vi "WeatherReport.vi"() -> ()   [LabVIEW 2016, in "WeatherReport.lvlib"]
doc: "This is a simple weather report which can display information for a particular day. This also has options to configure the properties of the controls"
uses:
  WeatherReport.lvlib
panel:
  in  "Settings":bool
  out "Humidity":string="40 %"
  out "Temperature":string="38°C "
  out "Weather":picture
  in  "Options":i32(listbox)
  in  "Stop":bool
  in  "Properties":string(tree)
  in  "Weather Report":i32(listbox)
  out "error out":errorcluster
  in  "Error In":errorcluster
  # "Overview: Demonstrates a typical weather report and provides options to configure the properties of these controls\nInstructions: \n1.Run the VI\n2.Select a particular day in the weather report\n3.The respective information of the day will be populated in the adjacent controls\n4.Click the settings option to list the configuration options for the controls\n5.Select a particular control's property, the possible options will be populated .\n6.Selecting an option applies the property to the control."
  # "The Properties are used to visualize the available controls and configure the visibility and accessibility of them. Selecting the Options applies the property to that control"
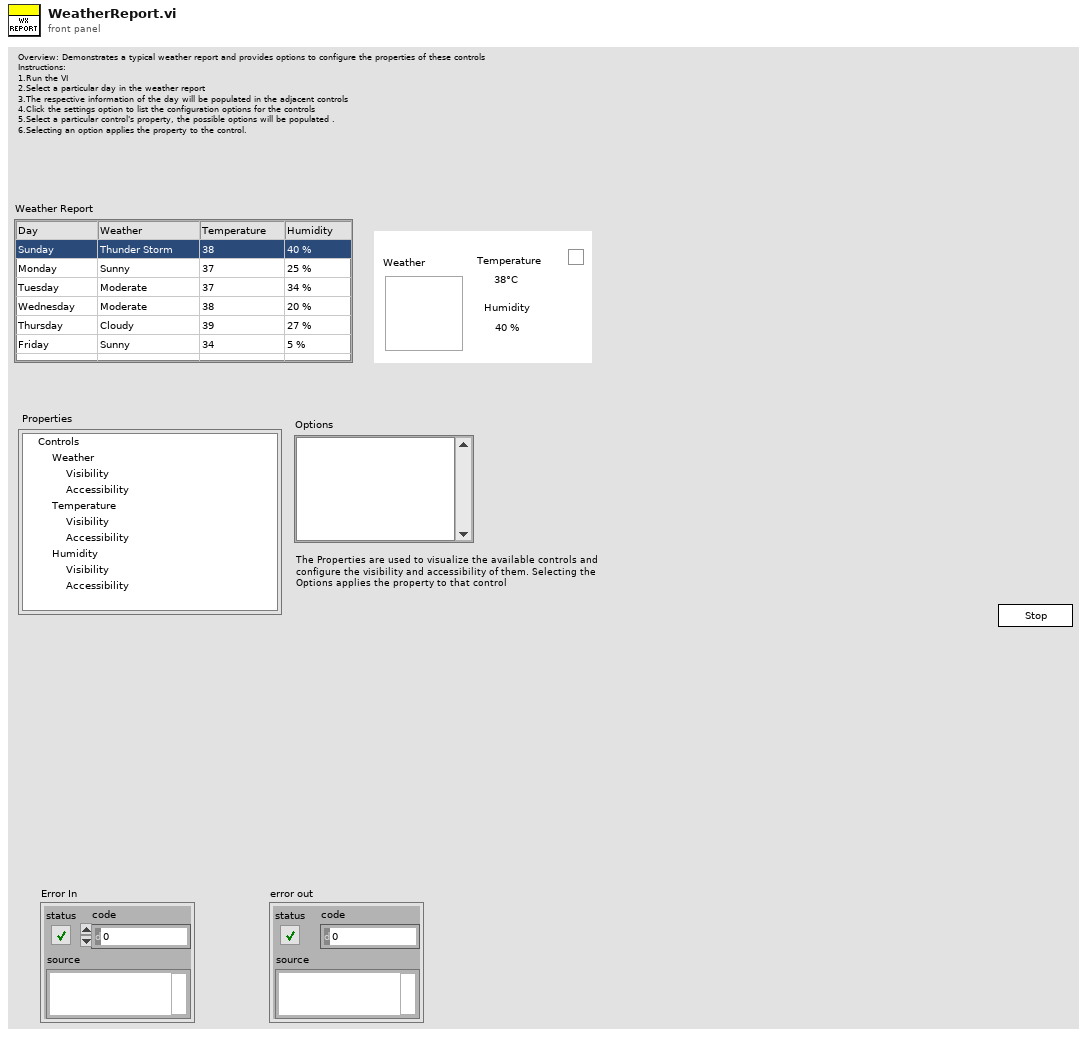
[diagram p1: front panel]
types:
  T1 = cluster{"Left":i16, "Top":i16, "Right":i16, "Bottom":i16}
  T2 = enum32{"Invalid", "Standard", "Closed", "Hidden", "Minimized", "Maximized"}
  T3 = enum32{"invalid app kind", "Development System", "Run Time System", "Student Edition", "Embedded LabVIEW", "Evaluation", "Custom"}
  T4 = enum8{"Enabled", "Disabled", "Disabled and Grayed Out"}
  T5 = enum8{"Enabled", "Disabled", "Disabled and Grayed Out"}[]
  T6 = cluster{"Core":cluster{"Current VI Reference":refnum<vi>, "Close Panel on Exit?":bool}, "Property":string, "Accessibility Array":i32[], "Visibility Array":i32[]}
  T7 = cluster{"Current VI Reference":refnum<vi>, "Close Panel on Exit?":bool}
  T8 = typedef "imagedata.ctl" = cluster{"image type":i32, "image depth":i32, "image":u8[], "mask":u8[], "colors":u32[], "Rectangle":cluster{"left":i16, "top":i16, "right":i16, "bottom":i16}}
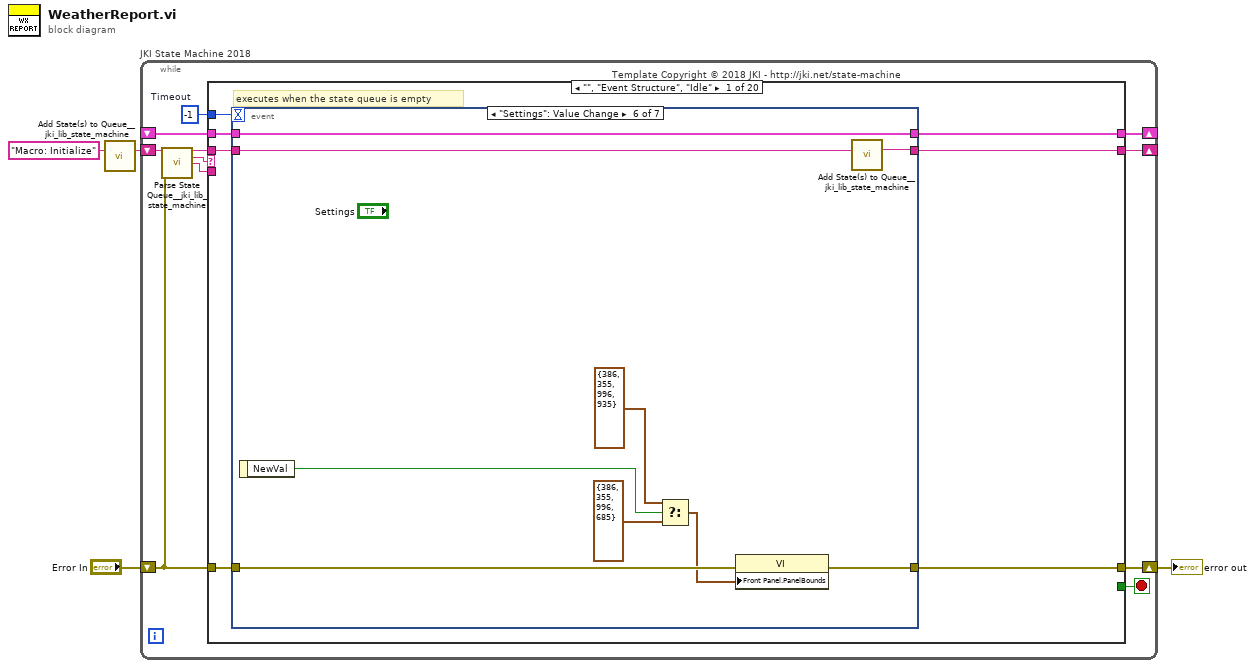
[diagram p0: block diagram]
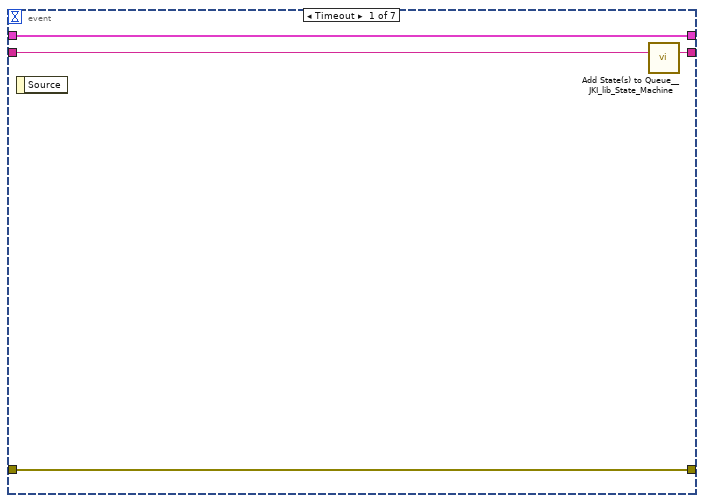
[diagram p2: hidden frame]
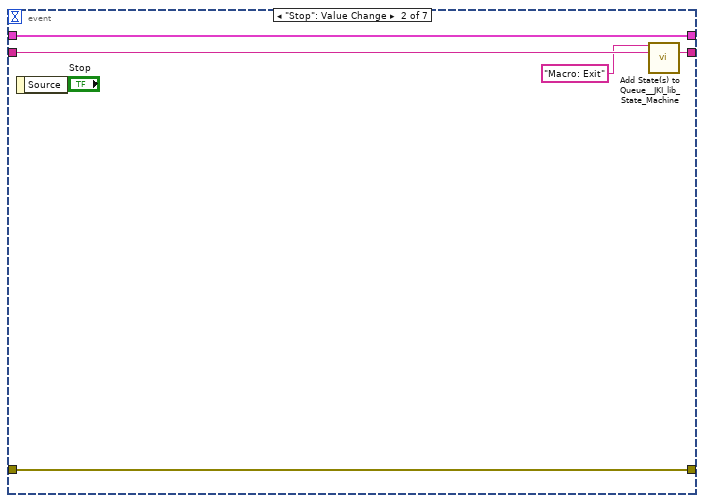
[diagram p3: hidden frame]
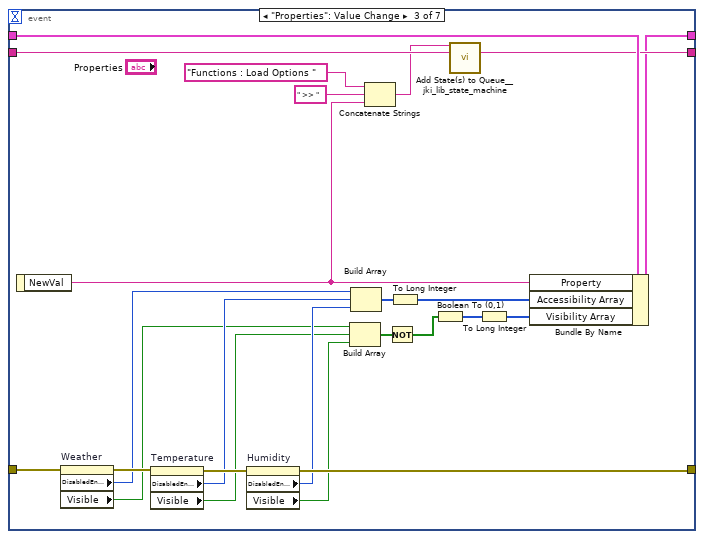
[diagram p4: hidden frame]
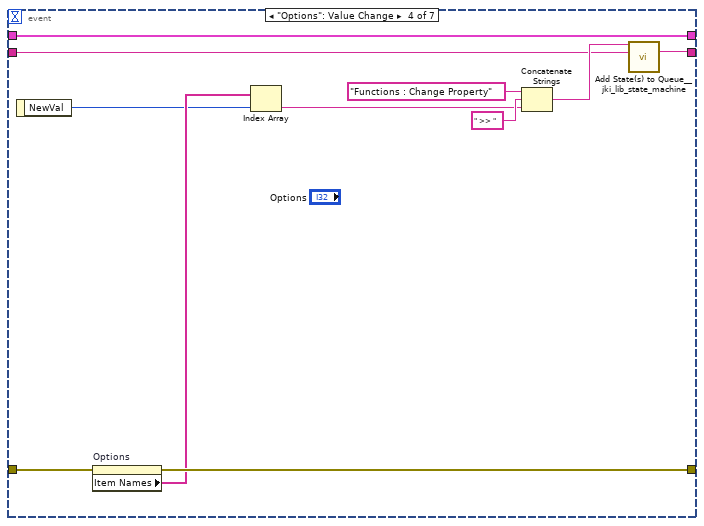
[diagram p5: hidden frame]
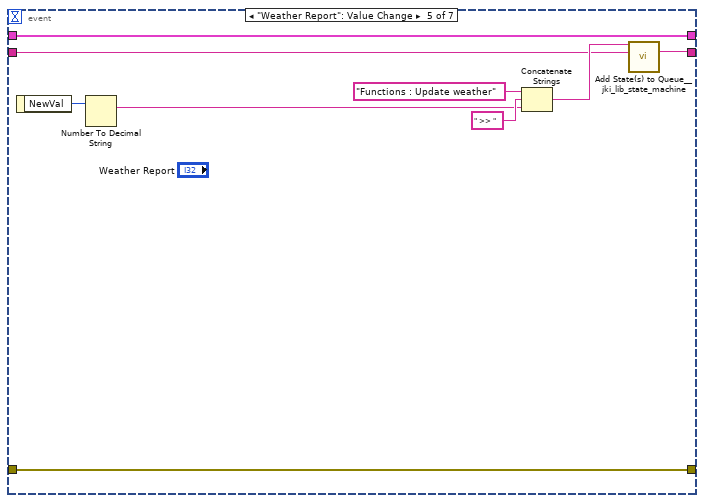
[diagram p6: hidden frame]
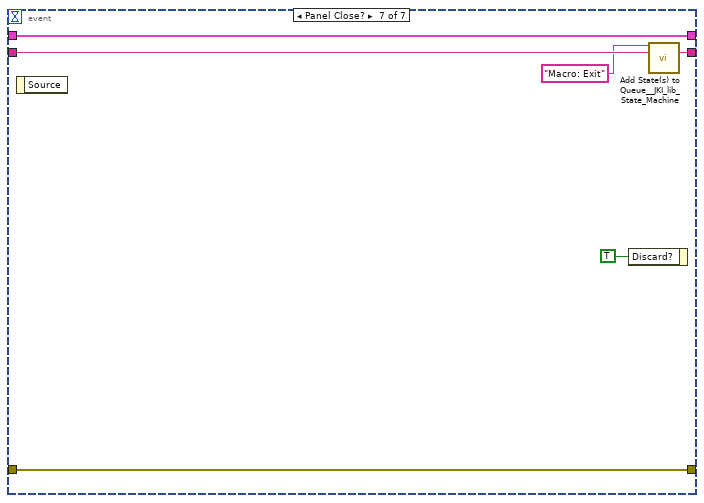
[diagram p7: hidden frame]
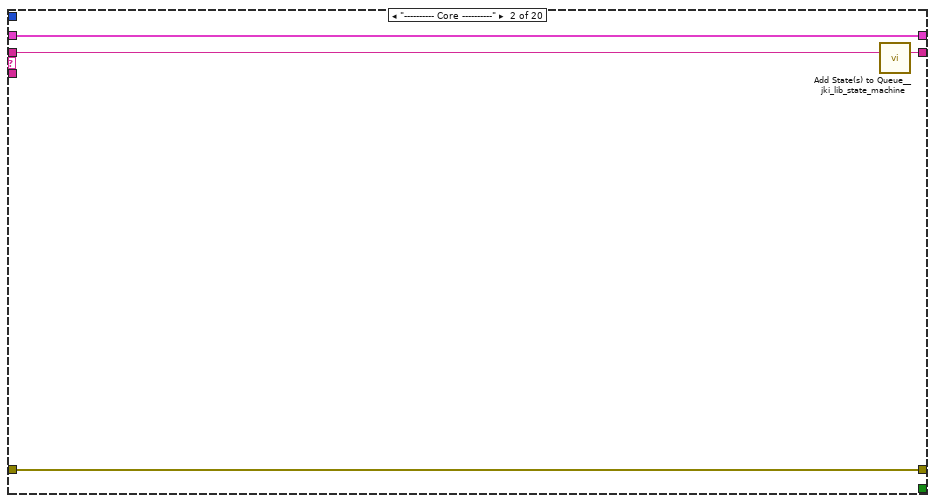
[diagram p8: hidden frame]
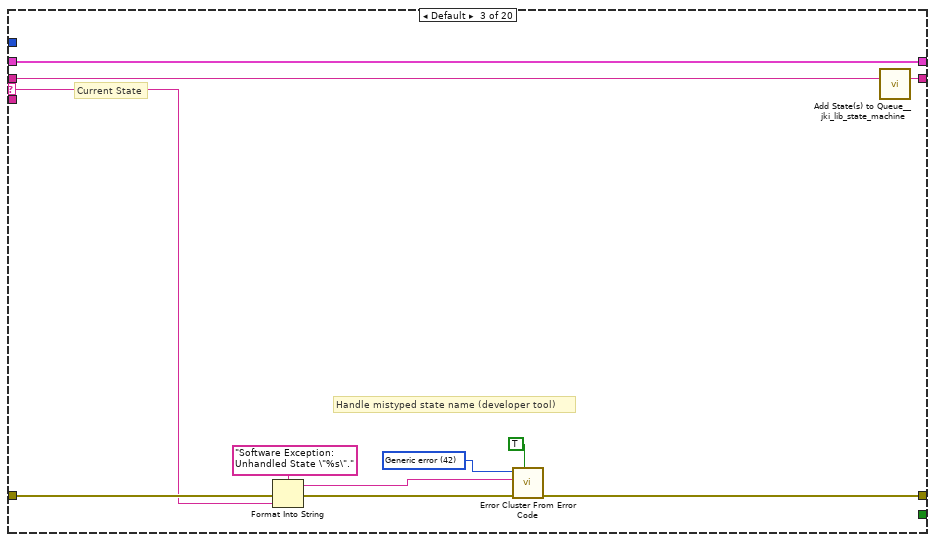
[diagram p9: hidden frame]
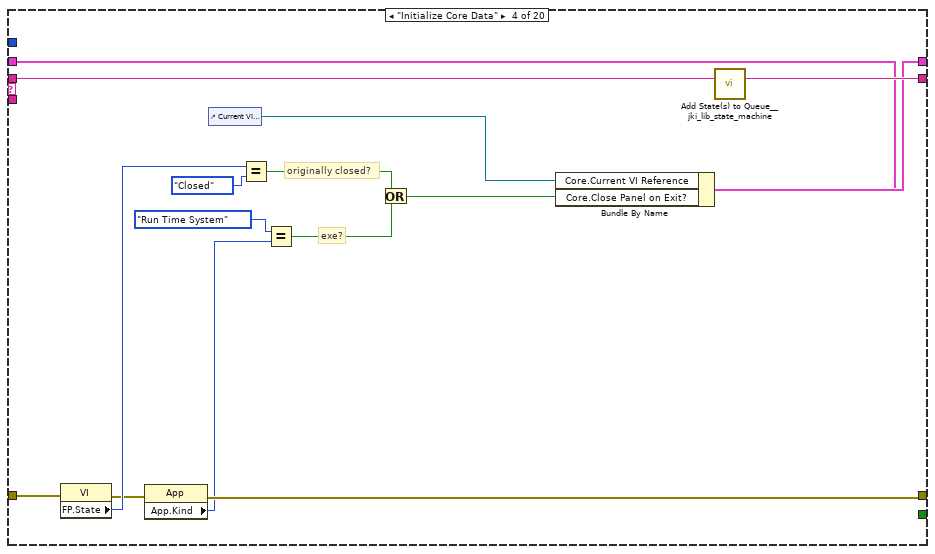
[diagram p10: hidden frame]
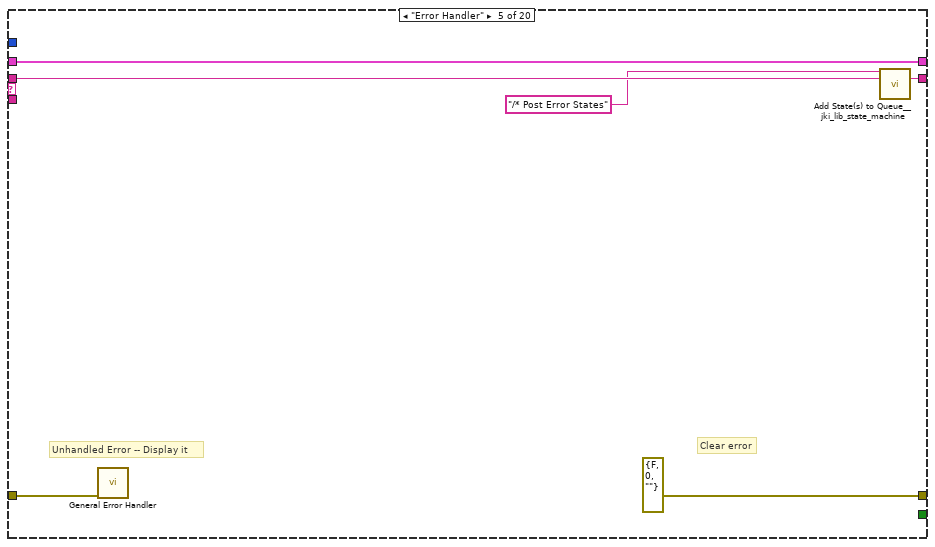
[diagram p11: hidden frame]
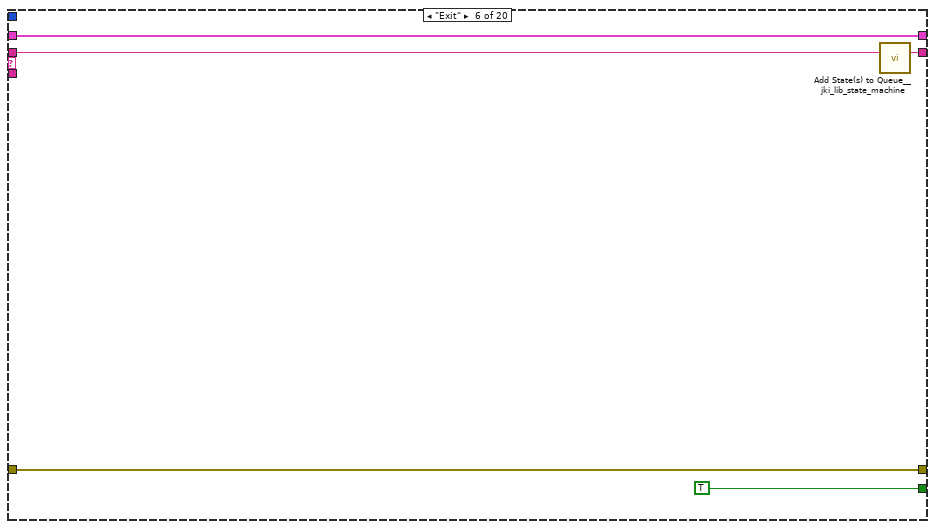
[diagram p12: hidden frame]
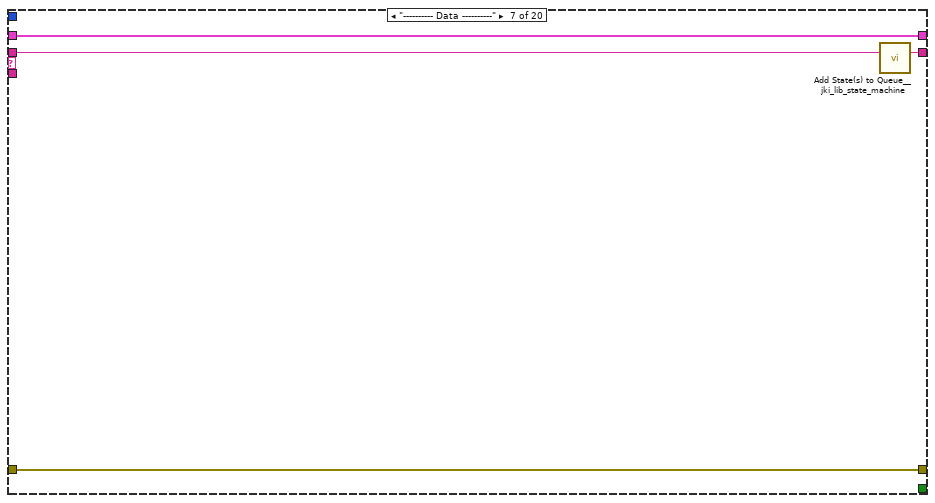
[diagram p13: hidden frame]
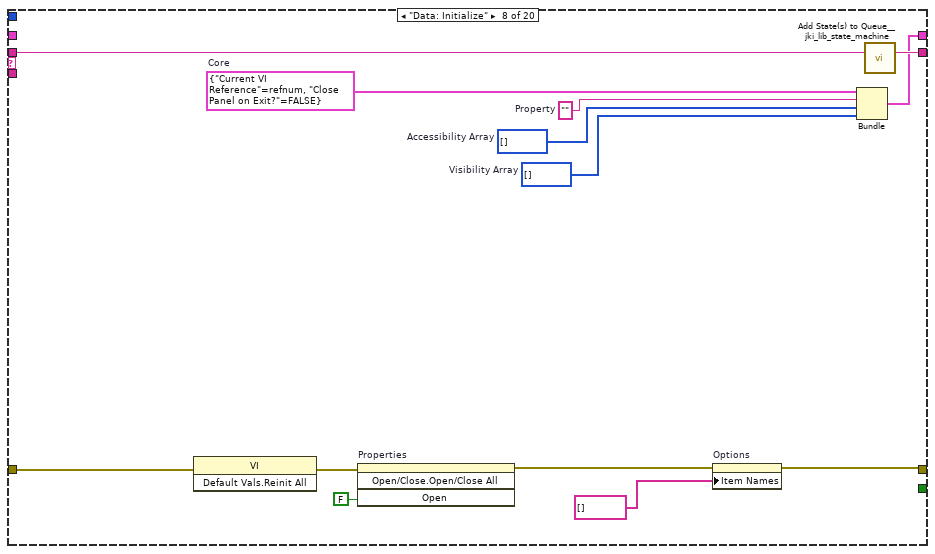
[diagram p14: hidden frame]
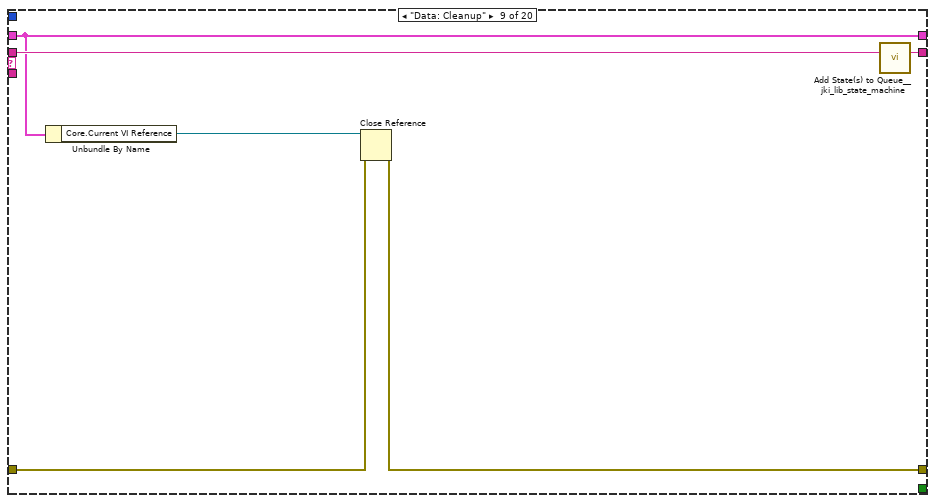
[diagram p15: hidden frame]
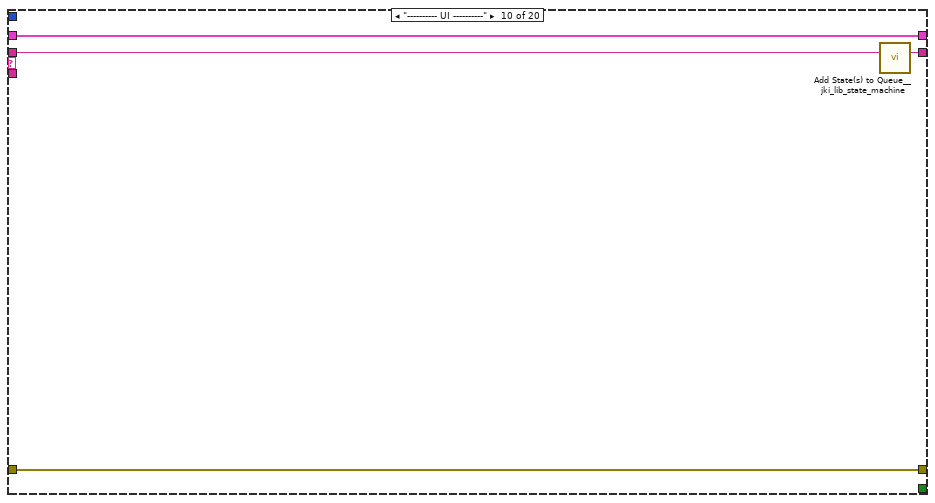
[diagram p16: hidden frame]
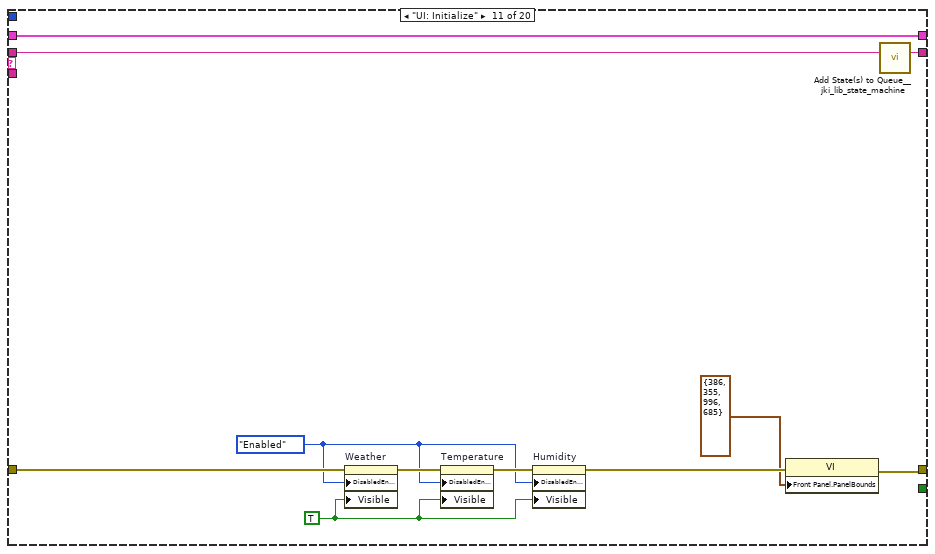
[diagram p17: hidden frame]
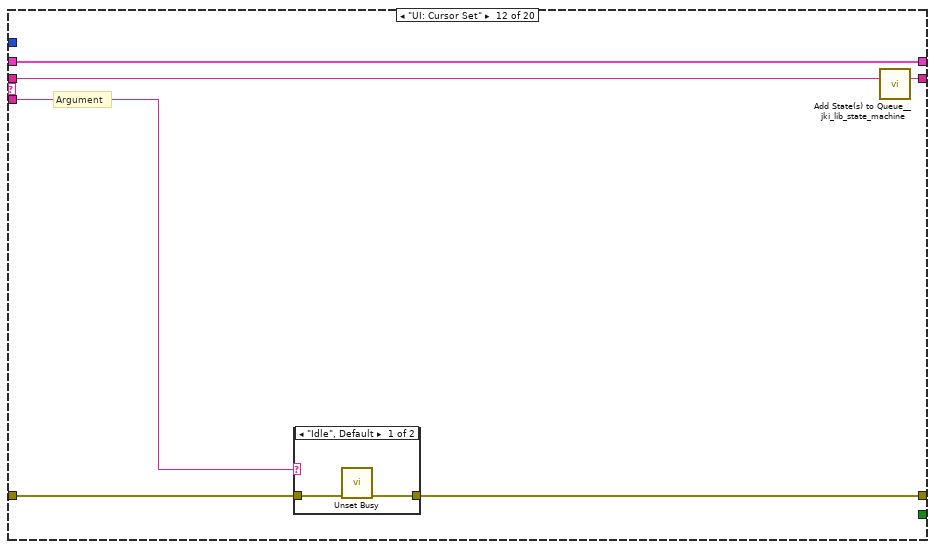
[diagram p18: hidden frame]
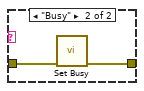
[diagram p19: hidden frame]
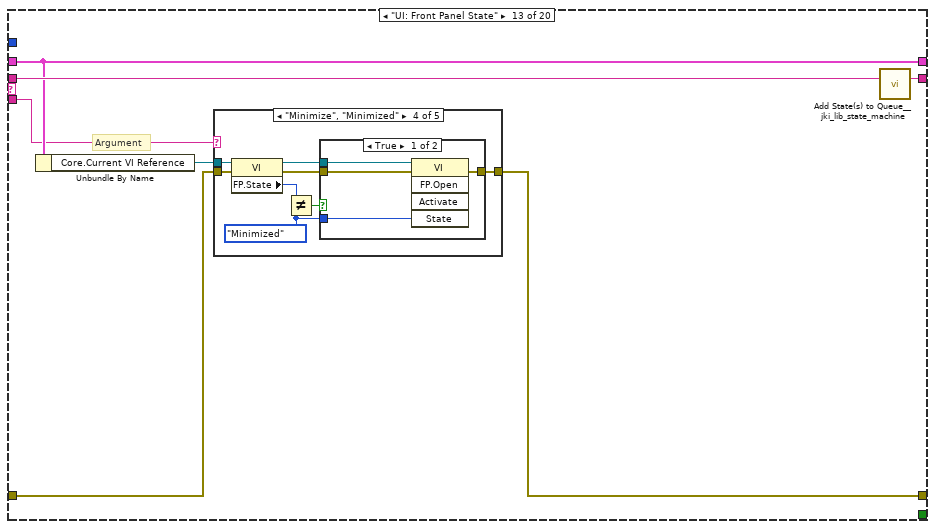
[diagram p20: hidden frame]
diagram:
  n1 = call <vilib>:"Add State(s) to Queue__jki_lib_state_machine.vi"("State(s) in (\"\")"="Macro: Initialize") -> ("States Out"=w4:string)  [unwired: 14 in]
  n2 = while "JKI State Machine 2018" {
    shift-right: [w8] -> _
    shift-left: _ -> [w7]
    shift-right: [w11] -> w1
    shift-left: "Error In" -> [w5]
    shift-right: [w10] -> _
    shift-left: w4 -> [w12]
    stop <- w9 stop-if-true
    w6 = -1  # Timeout
    # "Template Copyright © 2018 JKI - http://jki.net/state-machine"
    n3 = call <vilib>:"Parse State Queue__jki_lib_state_machine.vi"("State Queue"=w12, "Error In (no error)"=w5) -> ("Remaining States"=w14:string, "Current State"=w15:string, "Arguments"=w13:string)  [unwired: 11 in]
    n4 = case shown="\"\", \"Event Structure\", \"Idle\"" w15 {
      selector: w15 -> [_ _ w95 _ _ _ _ _ _ _ _ _ _ _ _ _ _ _ _ _]
      tunnel: w14 -> [w22 w94 w99 w120 w126 w131 w135 w148 w154 w158 w169 w175 w186 w255 w260 w270 w274 w293 w315 w366]
      tunnel: w13 -> [_ _ _ _ _ _ _ _ _ _ _ w170 w180 _ _ _ _ w281 w310 w354]
      tunnel: w7 -> [w20 w91 w97 w116 w123 w129 w132 _ w149 w155 w167 w173 w182 w252 w257 w267 w271 w285 w312 w364]
      tunnel: [w19 w92 w101 w107 errorcluster {"status"=FALSE, "code"=0, "source"=""} ("error out") w128 w133 w137 w150 w156 w163 w171 w183 w253 w258 w268 w272 w290 w303 w359] -> w11
      tunnel: w5 -> [w18 w92 w100 w110 w122 w128 w133 w143 w151 w156 w166 w172 w184 w253 w258 w268 w272 w291 w304 w360]
      tunnel: [w21 w93 w98 w119 w125 w130 w134 w147 w153 w157 w168 w174 w185 w254 w259 w269 w273 w292 w314 w365] -> w10
      tunnel: [_ _ _ _ _ TRUE _ _ _ _ _ _ _ _ _ _ _ _ _ _] -> w9
      tunnel: [w17 w91 w97 w118 w123 w129 w132 w146 w149 w155 w167 w173 w182 w252 w257 w267 w271 w285 w312 w364] -> w8
      tunnel: w6 -> [w16 _ _ _ _ _ _ _ _ _ _ _ _ _ _ _ _ _ _ _]
      frame "", "Event Structure", "Idle" {
        # "executes when the state queue is empty"
        n5 = event shown="[5] \"Settings\": Value Change" {
          selector: _ -> [_ _ _ _ _ _ _]
          dyn-events: _ -> [_ _ _ _ _ _ _]
          timeout: w16 -> [_ _ _ _ _ _ _]
          tunnel: w22 -> [w26 w31 w53 w61 w69 w82 w90]
          tunnel: [w25 w30 w52 w60 w68 w81 w89] -> w21
          tunnel: w20 -> [w23 w28 w54 w65 w74 w83 w87]
          tunnel: [w24 w29 w44 w59 w75 w80 w88] -> w19
          tunnel: w18 -> [w24 w29 w55 w66 w75 w84 w88]
          tunnel: [w23 w28 w48 w65 w74 w83 w87] -> w17
          event Timeout {
            n6 = event-data() -> ()  [unwired: 1 in, 1 out]
            n7 = call <vilib>:"Add State(s) to Queue__JKI_lib_State_Machine.vi"("State(s) in (\"\")"=w26) -> ("States Out"=w25:string)  [unwired: 14 in]
          }
          event "Stop": Value Change {
            n8 = event-data() -> ()  [unwired: 1 in, 1 out]
            n9 = call <vilib>:"Add State(s) to Queue__JKI_lib_State_Machine.vi"("State(s) in Front (\"\")"="Macro: Exit", "State(s) in (\"\")"=w31) -> ("States Out"=w30:string)  [unwired: 13 in]
          }
          event "Properties": Value Change {
            n10 = event-data() -> ("NewVal"=w47:string)  [unwired: 1 in]
            n11 = property on="Weather" class="Pict"(error in=w55) -> (error out=w46:errorcluster, "DisabledEnum"=w43:T4, "Visible"=w40:bool)  [unwired: 1 in, 1 out]
            n12 = property on="Temperature" class="Str"(error in=w46) -> (error out=w45:errorcluster, "DisabledEnum"=w42:T4, "Visible"=w39:bool)  [unwired: 1 in, 1 out]
            n13 = property on="Humidity" class="Str"(error in=w45) -> (error out=w44:errorcluster, "DisabledEnum"=w41:T4, "Visible"=w38:bool)  [unwired: 1 in, 1 out]
            n14 = Build Array(w40, w39, w38) -> (w33:bool[])
            n15 = Build Array(w43, w42, w41) -> (w37:T5)
            n16 = Concatenate Strings("Functions : Load Options " ("State(s) in Front (\"\")"), " >> " ("string"), w47) -> (w49:string)
            n17 = Not(x=w33) -> (.not. x?=w32:bool[])
            n18 = To Long Integer(number=w37) -> (32bit integer=w36:i32[])
            n19 = Boolean To (0,1)(Boolean=w32) -> (0, 1=w35:i16[])
            n20 = call <vilib>:"Add State(s) to Queue__jki_lib_state_machine.vi"("State(s) in Front (\"\")"=w49, "State(s) in (\"\")"=w53) -> ("States Out"=w52:string)  [unwired: 13 in]
            n21 = To Long Integer(number=w35) -> (32bit integer=w34:i32[])
            n22 = Bundle By Name(cluster=w54, "Property"=w47, "Accessibility Array"=w36, "Visibility Array"=w34) -> (w48:T6)
          }
          event "Options": Value Change {
            n23 = event-data() -> ("NewVal"=w57:i32)  [unwired: 1 in]
            n24 = property on="Options" class="LstBox (strict)"(error in=w66) -> (error out=w59:errorcluster, "Item Names"=w58:string[])  [unwired: 1 in, 1 out]
            n25 = Index Array(array=w58, index=w57) -> (element=w56:string)
            n26 = Concatenate Strings("Functions : Change Property" ("State(s) in Front (\"\")"), " >> " ("string"), w56) -> (w62:string)
            n27 = call <vilib>:"Add State(s) to Queue__jki_lib_state_machine.vi"("State(s) in Front (\"\")"=w62, "State(s) in (\"\")"=w61) -> ("States Out"=w60:string)  [unwired: 13 in]
          }
          event "Weather Report": Value Change {
            n28 = event-data() -> ("NewVal"=w73:i32)  [unwired: 1 in]
            n29 = Number To Decimal String(number=w73) -> (decimal integer string=w67:string)  [unwired: 1 in]
            n30 = Concatenate Strings("Functions : Update weather" ("State(s) in Front (\"\")"), " >> " ("string"), w67) -> (w70:string)
            n31 = call <vilib>:"Add State(s) to Queue__jki_lib_state_machine.vi"("State(s) in Front (\"\")"=w70, "State(s) in (\"\")"=w69) -> ("States Out"=w68:string)  [unwired: 13 in]
          }
          event "Settings": Value Change {
            n32 = event-data() -> ("NewVal"=w79:bool)  [unwired: 1 in]
            n33 = Select(t=T1 {"Left"=386, "Top"=355, "Right"=996, "Bottom"=935} ("Front Panel.PanelBounds"), s=w79, f=T1 {"Left"=386, "Top"=355, "Right"=996, "Bottom"=685} ("Front Panel.PanelBounds")) -> (s? t:f=w77:T1)
            n34 = property class="VI"(error in=w84, "Front Panel.PanelBounds"=w77) -> (error out=w80:errorcluster)  [unwired: 1 in, 1 out]
            n35 = call <vilib>:"Add State(s) to Queue__jki_lib_state_machine.vi"("State(s) in (\"\")"=w82) -> ("States Out"=w81:string)  [unwired: 14 in]
          }
          event Panel Close? {
            n36 = event-data() -> ()  [unwired: 1 in, 1 out]
            n37 = event-data("Discard?"=TRUE) -> ()  [unwired: 1 in, 1 out]
            n38 = call <vilib>:"Add State(s) to Queue__JKI_lib_State_Machine.vi"("State(s) in Front (\"\")"="Macro: Exit", "State(s) in (\"\")"=w90) -> ("States Out"=w89:string)  [unwired: 13 in]
          }
        }
      }
      frame "---------- Core ----------" {
        n39 = call <vilib>:"Add State(s) to Queue__jki_lib_state_machine.vi"("State(s) in (\"\")"=w94) -> ("States Out"=w93:string)  [unwired: 14 in]
      }
      frame Default {
        w104 = 42 items=["No error", "Argument error", "Memory is full", "Out of zone", "End of file", "File already open", "Generic file I/O error", "File not found", "File permission error", "Disk is full", "Duplicate path", "Too many files open", "System feature not enabled", "Resource file not found", "Cannot add resource", "Resource not found", "Image not found", "Image memory error", "Pen does not exist", "Config type invalid", "Config token not found", "Config parse error", "Config memory error", "Bad external code format", "Bad external code offset", "External code not present", "Null window", "Destroy window error", "Null menu", "Print aborted", "Bad print record", "Print driver error", "Windows error during printing", "Memory error during printing", "Print dialog error", "Generic print error", "Invalid device refnum", "Device not found", "Device parameter error", "Device unit error", "Cannot open device", "Device call aborted", "Generic error", "Cancelled by user", "Object ID too low", "Object ID too high", "Object not in heap", "Unknown heap", "Unknown object (invalid DefProc)", "Unknown object (DefProc not in table)", "Message out of range", "Invalid (null) method", "Unknown message", "Manager call not supported", "Bad address", "Network operation in progress", "Network operation timed out", "Connection is busy", "Network attribute not supported", "Network error", "Address in use", "System out of memory", "Connection aborted", "Connection refused", "Not connected", "Already connected", "Connection closed", "Initialization error (interapplication manager)", "Bad occurrence", "Wait on unbound occurrence handler", "Occurrence queue overflow", "Datalog type conflict", "Unused", "Unrecognized type (interapplication manager)", "Memory corrupt", "Failed to make temporary DLL", "Old CIN version", "Drag socket not found", "Failed to load drop-object", "Failed to register OLE object", "Failed to release OLE object", "Format specifier type mismatch", "Unknown format specifier", "Too few format specifiers", "Too many format specifiers", "Scan failed", "Newer CIN version", "Error converting to variant", "Runtime menu error", "Password tampered", "Variant attribute not found", "Incompatible variant data type", "Event data is not available", "Event Store is not present", "Occurrence is not found", "Event Queue is not created", "Event info is not available", "Refnum passed is NULL", "Error retrieving Class GUID", "Error retrieving CoClass GUID", "Error retrieving TypeLib GUID.", "Bad built application magic bytes.", "Specific driver is different from the specific driver associated with the Logical Name.", "There is no session opened to the class driver.", "Max Error", "MAX - Error with config objects", "MAX - Error loading configuration", "MAX - Group not supported"]
        # "Current State"
        # "Handle mistyped state name (developer tool)"
        n40 = Format Into String(format string="Software Exception: Unhandled State \"%s\"." ("message"), error in=w100, w95) -> (resulting string=w103:string, error out=w102:errorcluster)  [unwired: 1 in]
        n41 = call <vilib>:"Error Cluster From Error Code.vi"("show call chain? (False)"=TRUE, "error in (no error)"=w102, "error message (\"\")"=w103, "error code (0)"=w104) -> ("error out"=w101:errorcluster)  [unwired: 5 in]
        n42 = call <vilib>:"Add State(s) to Queue__jki_lib_state_machine.vi"("State(s) in (\"\")"=w99) -> ("States Out"=w98:string)  [unwired: 14 in]
      }
      frame "Initialize Core Data" {
        # "originally closed?"
        # "exe?"
        n43 = property class="VI"(error in=w110) -> (error out=w108:errorcluster, "FP.State"=w114:T2)  [unwired: 1 in, 1 out]
        n44 = property class="App"(error in=w108) -> (error out=w107:errorcluster, "App.Kind"=w106:T3)  [unwired: 1 in, 1 out]
        n45 = control-ref of="Current VI Reference"() -> (w111:refnum<vi>)
        n46 = Equal?(x=w114, y=T2."Closed" ("Front Panel Window:State")) -> (x = y?=w112:bool)
        n47 = Equal?(x=T3."Run Time System" ("Application:Kind"), y=w106) -> (x = y?=w117:bool)
        n48 = Or(x=w112, y=w117) -> (x .or. y?=w115:bool)
        n49 = Bundle By Name(cluster=w116, "Core.Current VI Reference"=w111, "Core.Close Panel on Exit?"=w115) -> (w118:T6)
        n50 = call <vilib>:"Add State(s) to Queue__jki_lib_state_machine.vi"("State(s) in (\"\")"=w120) -> ("States Out"=w119:string)  [unwired: 14 in]
      }
      frame "Error Handler" {
        # "Unhandled Error -- Display it"
        # "Clear error"
        n51 = call <vilib>:"General Error Handler.vi"("error in (no error)"=w122) -> ()  [unwired: 10 in, 5 out]
        n52 = call <vilib>:"Add State(s) to Queue__jki_lib_state_machine.vi"("State(s) in Front (\"\")"="/* Post Error States", "State(s) in (\"\")"=w126) -> ("States Out"=w125:string)  [unwired: 13 in]
      }
      frame "Exit" {
        n53 = call <vilib>:"Add State(s) to Queue__jki_lib_state_machine.vi"("State(s) in (\"\")"=w131) -> ("States Out"=w130:string)  [unwired: 14 in]
      }
      frame "---------- Data ----------" {
        n54 = call <vilib>:"Add State(s) to Queue__jki_lib_state_machine.vi"("State(s) in (\"\")"=w135) -> ("States Out"=w134:string)  [unwired: 14 in]
      }
      frame "Data: Initialize" {
        w141 = i32[] []  # Visibility Array
        w142 = i32[] []  # Accessibility Array
        w144 = T7 {"Current VI Reference"=refnum, "Close Panel on Exit?"=FALSE}  # Core
        w145 = ""  # Property
        n55 = invoke class="VI" method="Default Vals.Reinit All"(error in=w143) -> (error out=w140:errorcluster)  [unwired: 2 in, 2 out]
        n56 = invoke on="Properties" class="Tree (strict)" method="Open/Close.Open/Close All"(error in=w140, "Open"=FALSE ("Open?")) -> (error out=w139:errorcluster)  [unwired: 2 in, 3 out]
        n57 = property on="Options" class="LstBox (strict)"(error in=w139, "Item Names"=string[] []) -> (error out=w137:errorcluster)  [unwired: 1 in, 1 out]
        n58 = Bundle("Core"=w144, "Property"=w145, "Accessibility Array"=w142, "Visibility Array"=w141) -> (w146:T6)  [unwired: 1 in]
        n59 = call <vilib>:"Add State(s) to Queue__jki_lib_state_machine.vi"("State(s) in (\"\")"=w148) -> ("States Out"=w147:string)  [unwired: 14 in]
      }
      frame "Data: Cleanup" {
        n60 = Unbundle By Name(w149) -> ("Core.Current VI Reference"=w152:refnum<vi>)
        n61 = Close Reference(reference=w152, error in (no error)=w151) -> (error out=w150:errorcluster)
        n62 = call <vilib>:"Add State(s) to Queue__jki_lib_state_machine.vi"("State(s) in (\"\")"=w154) -> ("States Out"=w153:string)  [unwired: 14 in]
      }
      frame "---------- UI ----------" {
        n63 = call <vilib>:"Add State(s) to Queue__jki_lib_state_machine.vi"("State(s) in (\"\")"=w158) -> ("States Out"=w157:string)  [unwired: 14 in]
      }
      frame "UI: Initialize" {
        w160 = TRUE ("Visible")
        w161 = T4."Enabled" ("Disabled")
        n64 = property on="Weather" class="Pict"(error in=w166, "DisabledEnum"=w161, "Visible"=w160) -> (error out=w165:errorcluster)  [unwired: 1 in, 1 out]
        n65 = property on="Temperature" class="Str"(error in=w165, "DisabledEnum"=w161, "Visible"=w160) -> (error out=w164:errorcluster)  [unwired: 1 in, 1 out]
        n66 = property on="Humidity" class="Str"(error in=w164, "DisabledEnum"=w161, "Visible"=w160) -> (error out=w162:errorcluster)  [unwired: 1 in, 1 out]
        n67 = property class="VI"(error in=w162, "Front Panel.PanelBounds"=T1 {"Left"=386, "Top"=355, "Right"=996, "Bottom"=685}) -> (error out=w163:errorcluster)  [unwired: 1 in, 1 out]
        n68 = call <vilib>:"Add State(s) to Queue__jki_lib_state_machine.vi"("State(s) in (\"\")"=w169) -> ("States Out"=w168:string)  [unwired: 14 in]
      }
      frame "UI: Cursor Set" {
        # "Argument"
        n69 = case shown="\"Idle\", Default" w170 {
          tunnel: w172 -> [w177 w179]
          tunnel: [w176 w178] -> w171
          frame "Idle", Default {
            n70 = call <vilib>:"Unset Busy.vi"("error in (no error)"=w177) -> ("error out"=w176:errorcluster)  [unwired: 10 in]
          }
          frame "Busy" {
            n71 = call <vilib>:"Set Busy.vi"("error in (no error)"=w179) -> ("error out"=w178:errorcluster)  [unwired: 9 in, 1 out]
          }
        }
        n72 = call <vilib>:"Add State(s) to Queue__jki_lib_state_machine.vi"("State(s) in (\"\")"=w175) -> ("States Out"=w174:string)  [unwired: 14 in]
      }
      frame "UI: Front Panel State" {
        # "Argument"
        n73 = Unbundle By Name(w182) -> ("Core.Current VI Reference"=w181:refnum<vi>)
        n74 = case shown="\"Minimize\", \"Minimized\"" w180 {
          tunnel: w184 -> [w192 w207 w218 w231 w244]
          tunnel: [w194 w208 w220 w233 w246] -> w183
          tunnel: w181 -> [w193 w205 w219 w232 w245]
          frame "Open", "Standard", Default {
            w187 = T2."Standard" ("State")
            n75 = property class="VI"(reference=w193, error in=w192) -> (reference out=w190:refnum<vi>, error out=w191:errorcluster, "FP.State"=w189:T2)
            n76 = Not Equal?(x=w189, y=w187) -> (x != y?=w188:bool)
            n77 = case shown="True" w188 {
              tunnel: [w198 w200] -> w194
              tunnel: w191 -> [w197 w200]
              tunnel: w190 -> [w196 _]
              tunnel: w187 -> [w195 _]
              frame True {
                n78 = invoke class="VI" method="FP.Open"(reference=w196, error in=w197, "Activate"=TRUE, "State"=w195) -> (error out=w198:errorcluster)  [unwired: 1 in, 4 out]
              }
              frame False {
              }
            }
          }
          frame "Close", "Closed" {
            n79 = property class="VI"(reference=w205, error in=w207) -> (reference out=w204:refnum<vi>, error out=w206:errorcluster, "FP.State"=w202:T2)
            n80 = Not Equal?(x=w202, y=T2."Closed" ("Front Panel Window:State")) -> (x != y?=w201:bool)
            n81 = case shown="True" w201 {
              tunnel: [w209 w212] -> w208
              tunnel: w206 -> [w209 w211]
              tunnel: w204 -> [_ w210]
              frame False {
              }
              frame True {
                n82 = invoke class="VI" method="FP.Close"(reference=w210, error in=w211) -> (error out=w212:errorcluster)  [unwired: 1 in, 2 out]
              }
            }
          }
          frame "Hidden", "Hide" {
            w213 = T2."Hidden" ("State")
            n83 = property class="VI"(reference=w219, error in=w218) -> (reference out=w216:refnum<vi>, error out=w217:errorcluster, "FP.State"=w215:T2)
            n84 = Not Equal?(x=w215, y=w213) -> (x != y?=w214:bool)
            n85 = case shown="True" w214 {
              tunnel: [w224 w225] -> w220
              tunnel: w217 -> [w223 w225]
              tunnel: w216 -> [w222 _]
              tunnel: w213 -> [w221 _]
              frame True {
                n86 = invoke class="VI" method="FP.Open"(reference=w222, error in=w223, "State"=w221) -> (error out=w224:errorcluster)  [unwired: 2 in, 4 out]
              }
              frame False {
              }
            }
          }
          frame "Minimize", "Minimized" {
            w226 = T2."Minimized" ("State")
            n87 = property class="VI"(reference=w232, error in=w231) -> (reference out=w229:refnum<vi>, error out=w230:errorcluster, "FP.State"=w228:T2)
            n88 = Not Equal?(x=w228, y=w226) -> (x != y?=w227:bool)
            n89 = case shown="True" w227 {
              tunnel: [w237 w238] -> w233
              tunnel: w230 -> [w236 w238]
              tunnel: w229 -> [w235 _]
              tunnel: w226 -> [w234 _]
              frame True {
                n90 = invoke class="VI" method="FP.Open"(reference=w235, error in=w236, "State"=w234) -> (error out=w237:errorcluster)  [unwired: 2 in, 4 out]
              }
              frame False {
              }
            }
          }
          frame "Maximize", "Maximized" {
            w239 = T2."Maximized" ("State")
            n91 = property class="VI"(reference=w245, error in=w244) -> (reference out=w242:refnum<vi>, error out=w243:errorcluster, "FP.State"=w241:T2)
            n92 = Not Equal?(x=w241, y=w239) -> (x != y?=w240:bool)
            n93 = case shown="True" w240 {
              tunnel: [w250 w251] -> w246
              tunnel: w243 -> [w249 w251]
              tunnel: w242 -> [w248 _]
              tunnel: w239 -> [w247 _]
              frame True {
                n94 = invoke class="VI" method="FP.Open"(reference=w248, error in=w249, "State"=w247) -> (error out=w250:errorcluster)  [unwired: 2 in, 4 out]
              }
              frame False {
              }
            }
          }
        }
        n95 = call <vilib>:"Add State(s) to Queue__jki_lib_state_machine.vi"("State(s) in (\"\")"=w186) -> ("States Out"=w185:string)  [unwired: 14 in]
      }
      frame "---------- Macro ----------" {
        n96 = call <vilib>:"Add State(s) to Queue__jki_lib_state_machine.vi"("State(s) in (\"\")"=w255) -> ("States Out"=w254:string)  [unwired: 14 in]
      }
      frame "Macro: Initialize" {
        w256 = "Data: Initialize\nInitialize Core Data\nUI: Initialize\nUI: Front Panel State >> Open"  # Data: Initialize Initialize Core Data UI: Initialize UI: Front Panel State >> Open
        n97 = call <vilib>:"Add State(s) to Queue__jki_lib_state_machine.vi"("State(s) in Front (\"\")"=w256, "State(s) in (\"\")"=w260) -> ("States Out"=w259:string)  [unwired: 13 in]
      }
      frame "Macro: Exit" {
        n98 = Unbundle By Name(w267) -> ("Core.Close Panel on Exit?"=w266:bool)
        n99 = Select(t="UI: Front Panel State >> Close", s=w266, f="") -> (s? t:f=w263:string)
        n100 = call <vilib>:"Add State(s) to Queue__jki_lib_state_machine.vi"("State(s) in (\"\")"=w263, "State(s) at Back (\"\")"="Data: Cleanup\nExit") -> ("States Out"=w261:string)  [unwired: 13 in]
        n101 = call <vilib>:"Add State(s) to Queue__jki_lib_state_machine.vi"("State(s) in Front (\"\")"=w261, "State(s) in (\"\")"=w270) -> ("States Out"=w269:string)  [unwired: 13 in]
      }
      frame "---------- Functionality ----------" {
        n102 = call <vilib>:"Add State(s) to Queue__jki_lib_state_machine.vi"("State(s) in (\"\")"=w274) -> ("States Out"=w273:string)  [unwired: 14 in]
      }
      frame "Functions : Load Options" {
        n103 = Unbundle By Name(w285) -> ("Accessibility Array"=w284:i32[], "Visibility Array"=w283:i32[])
        n104 = String Length(string=w281) -> (length=w288:i32)
        n105 = case shown="\"Humidity\", \"Temperature\", \"Weather\", Default" w281 {
          tunnel: [string[] ["Enabled", "Disabled", "Disabled and greyed out"] ("Item Names") string[] ["Visible", "Invisible"] ("Item Names") string[] [] ("Item Names")] -> w289
          frame "Accessibility_0", "Accessibility_1", "Accessibility_2" {
          }
          frame "Visibility_0", "Visibility_1", "Visibility_2" {
          }
          frame "Humidity", "Temperature", "Weather", Default {
          }
        }
        n106 = Decrement(x=w288) -> (x-1=w287:i32)
        n107 = String Subset(string=w281, offset (0)=w287) -> (substring=w286:string)  [unwired: 1 in]
        n108 = Decimal String To Number(string=w286) -> (number=w282:i32)  [unwired: 2 in, 1 out]
        n109 = Index Array(array=w284, index=w282) -> (element=w277:i32)
        n110 = Index Array(array=w283, index=w282) -> (element=w276:i32)
        n111 = Match Pattern(string=w281, regular expression="Visibility") -> (offset past match=w279:i32)  [unwired: 1 in, 3 out]
        n112 = Less Than 0?(x=w279) -> (x < 0?=w278:bool)
        n113 = Select(t=w277, s=w278, f=w276) -> (s? t:f=w275:i32)
        n114 = property on="Options" class="LstBox (strict)"(error in=w291, "Item Names"=w289, "Value"=w275) -> (error out=w290:errorcluster)  [unwired: 1 in, 1 out]
        n115 = call <vilib>:"Add State(s) to Queue__jki_lib_state_machine.vi"("State(s) in (\"\")"=w293) -> ("States Out"=w292:string)  [unwired: 14 in]
      }
      frame "Functions : Change Property" {
        n116 = Unbundle By Name(w312) -> ("Property"=w311:string, "Accessibility Array"=w302:i32[], "Visibility Array"=w301:i32[])
        n117 = Match Pattern(string=w311, regular expression="_") -> (after substring=w305:string)  [unwired: 1 in, 3 out]
        n118 = Decimal String To Number(string=w305) -> (number=w300:i32)  [unwired: 2 in, 1 out]
        n119 = Index Array(array=w302, index=w300) -> (element=w309:i32)
        n120 = Index Array(array=w301, index=w300) -> (element=w307:i32)
        n121 = Equal To 0?(x=w307) -> (x = 0?=w297:bool)
        n122 = Type Cast(type=T4."Enabled" ("Disabled"), x=w309) -> (*(type *) &x=w306:T4)
        n123 = case shown="\"Disabled and greyed out\"" w310 {
          tunnel: [TRUE ("Visible") FALSE ("Visible") w333 w336 w338 w339] -> w299
          tunnel: [w329 w331 T4."Enabled" ("Disabled") T4."Disabled" ("Disabled") T4."Disabled and Grayed Out" ("Disabled") w340] -> w298
          tunnel: w297 -> [_ _ w333 w336 w338 w339]
          tunnel: w306 -> [w329 w331 _ _ _ w340]
          frame "Visible" {
          }
          frame "Invisible" {
          }
          frame "Enabled" {
          }
          frame "Disabled" {
          }
          frame "Disabled and greyed out" {
          }
          frame Default {
          }
        }
        n124 = case shown="\"0\"" w305 {
          tunnel: w304 -> [w319 w323 w327 w328]
          tunnel: [w318 w322 w326 w328] -> w303
          tunnel: w298 -> [w317 w321 w325 _]
          tunnel: w299 -> [w316 w320 w324 _]
          frame "0" {
            n125 = property on="Weather" class="Pict"(error in=w319, "DisabledEnum"=w317, "Visible"=w316) -> (error out=w318:errorcluster)  [unwired: 1 in, 1 out]
          }
          frame "1" {
            n126 = property on="Temperature" class="Str"(error in=w323, "DisabledEnum"=w321, "Visible"=w320) -> (error out=w322:errorcluster)  [unwired: 1 in, 1 out]
          }
          frame "2" {
            n127 = property on="Humidity" class="Str"(error in=w327, "DisabledEnum"=w325, "Visible"=w324) -> (error out=w326:errorcluster)  [unwired: 1 in, 1 out]
          }
          frame Default {
          }
        }
        n128 = call <vilib>:"Add State(s) to Queue__jki_lib_state_machine.vi"("State(s) in (\"\")"=w315) -> ("States Out"=w314:string)  [unwired: 14 in]
      }
      frame "Functions : Update weather" {
        n129 = property on="Weather Report" class="MCListbox (strict)"(error in=w360) -> (error out=w355:errorcluster, "ItemNames"=w353:string[][])  [unwired: 1 in, 1 out]
        n130 = Decimal String To Number(string=w354) -> (number=w342:i32)  [unwired: 2 in, 1 out]
        n131 = Index Array(array=w353, index (row) #1=w342, index (col) #1=1 ("disabled index (col)"), index (row) #2=w342, index (col) #2=2 ("disabled index (col)"), index (row) #3=w342, index (col) #3=3 ("disabled index (col)")) -> (element #1=w346:string, element #2=w351:string, element #3=→"Humidity":string)
        n132 = Concatenate Strings(w351, "°C" ("string")) -> (→"Temperature":string)
        n133 = Concatenate Strings("Images\\\\" ("string"), w346, ".png" ("string")) -> (w344:string)
        n134 = Current VI's Path() -> (path=w358:path)
        n135 = Strip Path(path=w358) -> (stripped path=w357:path)  [unwired: 1 out]
        n136 = Build Path(base path=w357, name or relative path=w344) -> (appended path=w356:path)
        n137 = call <vilib>:"Read PNG File.vi"("error in (no error)"=w355, "path to PNG file"=w356) -> ("error out"=w359:errorcluster, "image data"=w362:T8)  [unwired: 7 in, 1 out]
        n138 = call <vilib>:"Draw Flattened Pixmap.vi"("image data"=w362, "picture"=picture data[5B]) -> ("new picture"=→"Weather":picture)  [unwired: 7 in]
        n139 = call <vilib>:"Add State(s) to Queue__jki_lib_state_machine.vi"("State(s) in (\"\")"=w366) -> ("States Out"=w365:string)  [unwired: 14 in]
      }
    }
  }
  "error out" <- w1
